vi "Measure Current.vi"(0 "VISA resource name":refnum<visa-resource-name>, 11 "error in (no error)":errorcluster) -> (4 "VISA resource name out":refnum<visa-resource-name>, 6 "Measurement":dbl, 15 "error out":errorcluster)   [LabVIEW 2025, in "Keithley 648X Series.lvlib"]
doc: "Returns a fresh current measurement.\n\n<b>Note:</b>\nThe Arm Loop Count cannot be infinity when using this VI. Use the <b>Configure Arm</b> VI to set it to a proper number."
uses:
  Keithley 648X Series.lvlib
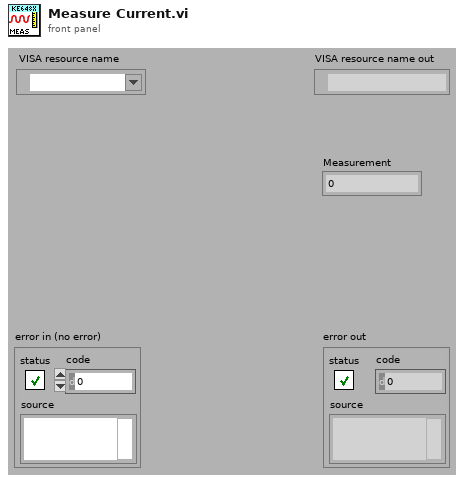
[diagram p1: front panel]
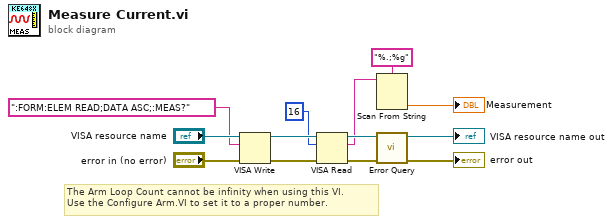
[diagram p0: block diagram]
diagram:
  # "The Arm Loop Count cannot be infinity when using this VI.\nUse the Configure Arm.VI to set it to a proper number."
  n1 = VISA Write(VISA resource name="VISA resource name", write buffer=":FORM:ELEM READ;DATA ASC;:MEAS?" ("Initiate"), error in (no error)="error in (no error)") -> (VISA resource name out=w10:refnum<visa-resource-name>, error out=w9:errorcluster)  [unwired: 1 out]
  n2 = VISA Read(VISA resource name=w10, byte count=u32 16, error in (no error)=w9) -> (VISA resource name out=w4:refnum<visa-resource-name>, read buffer=w1:string, error out=w5:errorcluster)  [unwired: 1 out]
  n3 = Scan From String(format string="%.;%g", input string=w1) -> (output 1=→"Measurement":dbl)  [unwired: 3 in, 3 out]
  n4 = call "Error Query.vi"("error in (no error)"=w5, "VISA resource name"=w4) -> ("error out"=→"error out":errorcluster, "VISA resource name out"=→"VISA resource name out":refnum<visa-resource-name>)  [unwired: 6 in, 2 out]
